vi "receive_one.vi"(8 "error in (no error)":errorcluster, 10 "Queue Name in":string, 11 "RabbitMQ Session In":T1) -> (0 "error out":errorcluster, 1 "Message out":string, 2 "Queue Name out":string, 3 "RabbitMQ Session Out":T1)   [LabVIEW 2019, in "rabbitmq.lvlib"]
uses:
  rabbitmq.lvlib
  session.ctl
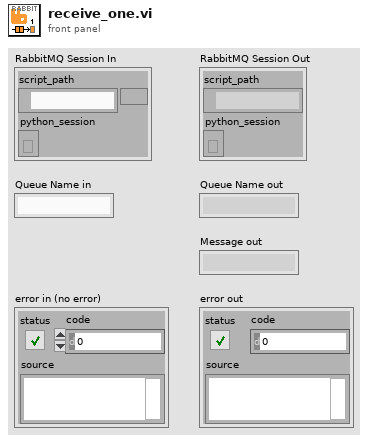
[diagram p1: front panel]
types:
  T1 = typedef "rabbitmq.lvlib/session.ctl" = cluster{"script_path":path, "python_session":refnum<k35>}
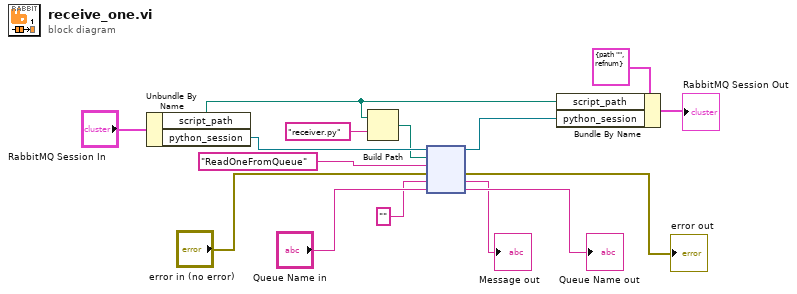
[diagram p0: block diagram]
diagram:
  n1 = Unbundle By Name("RabbitMQ Session In") -> ("script_path"=w4:path, "python_session"=w9:refnum<k35>)
  n2 = Build Path(base path=w4, name or relative path="receiver.py") -> (appended path=w3:path)
  n3 = node(w9, w3, "ReadOneFromQueue" ("function name"), "error in (no error)", "", "Queue Name in") -> (w15:refnum<k35>, →"error out":errorcluster, →"Message out":string, →"Queue Name out":string)  [unwired: 2 out]
  n4 = Bundle By Name(cluster=T1 {"script_path"=path "", "python_session"=refnum}, "script_path"=w4, "python_session"=w15) -> (→"RabbitMQ Session Out":T1)
